vi "Set Period.vi"(8 "error in (no error)":errorcluster, 10 "Period [ms]":i32, 11 "Actor API in":refnum<class "Metronome Actor API.lvclass">) -> (0 "error out":errorcluster)   [LabVIEW 2015, in "Metronome Actor API.lvclass"]
uses:
  Metronome Actor API.lvclass
  Messaging/Message/Message.lvclass/Message.ctl
  Messaging/Message/Message.lvclass
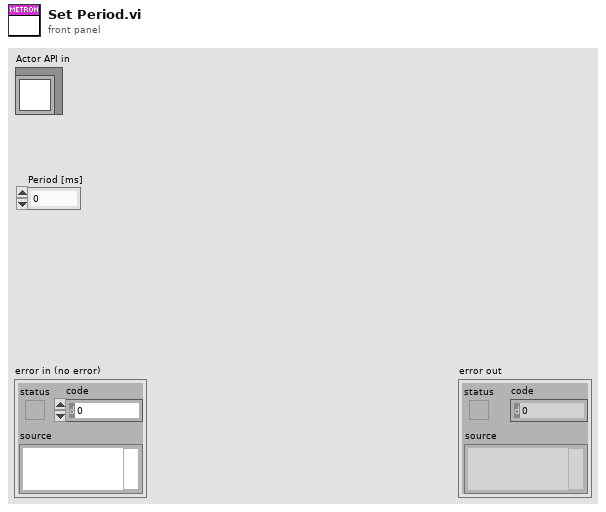
[diagram p1: front panel]
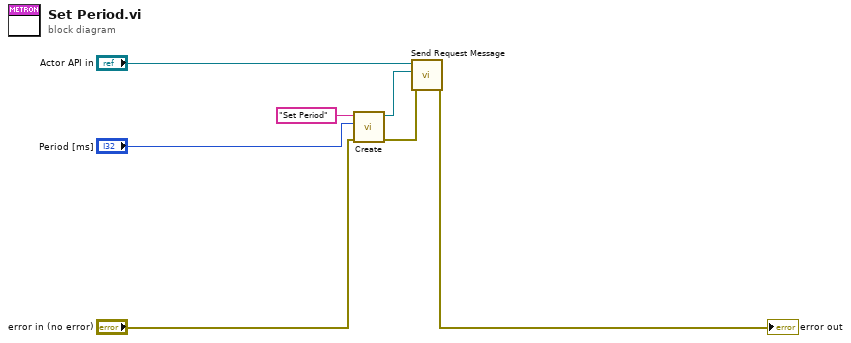
[diagram p0: block diagram]
diagram:
  n1 = call "Create.vi"("error in (no error)"="error in (no error)", "Data"="Period [ms]", "Name"="Set Period" ("Parameter")) -> ("error out"=w1:errorcluster, "Message out"=w2:refnum<class "Message.lvclass">)  [unwired: 7 in]
  n2 = call-dynamic "Send Request Message.vi"("error in (no error)"=w1, "Message"=w2, "Actor API in"="Actor API in") -> ("error out"=→"error out":errorcluster)  [unwired: 8 in]
